vi "errorHandling.vi"() -> ()   [LabVIEW 2014]
uses:
  <vilib>/gmath/statdist.llb/Normal PDF.vi
  <vilib>/gmath/statdist.llb/Poisson Random.vi
  <vilib>/gmath/NI_Gmath.lvlib
panel:
  in  "Normalization 3":dbl
  in  "Normalization 2":dbl
  in  "Normalization 1":dbl
  out "Error State":errorcluster
  out "Waveform Graph":i32[](graph)
  in  "Standard Dev. 3":dbl=5.0 format="%#_13g"
  in  "Mean 3":dbl=25.0 format="%#_13g"
  in  "Standard Dev. 2":dbl=5.0 format="%#_13g"
  in  "Mean 2":dbl=25.0 format="%#_13g"
  in  "Standard Dev. 1":dbl=5.0 format="%#_13g"
  in  "Mean 1":dbl=25.0 format="%#_13g"
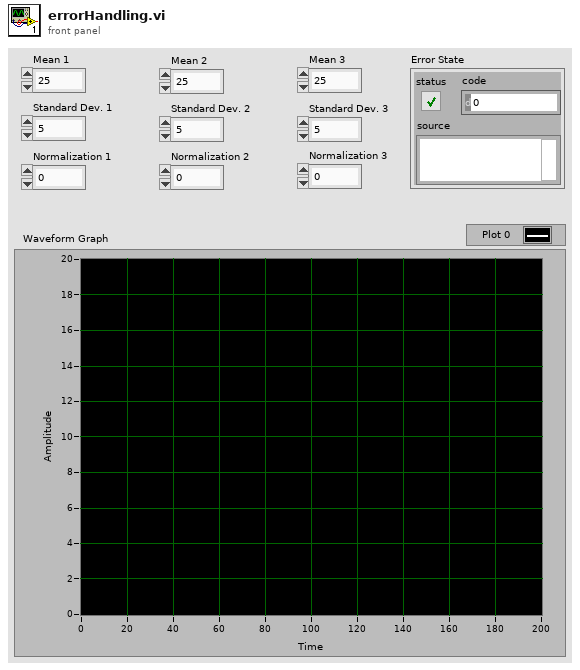
[diagram p1: front panel]
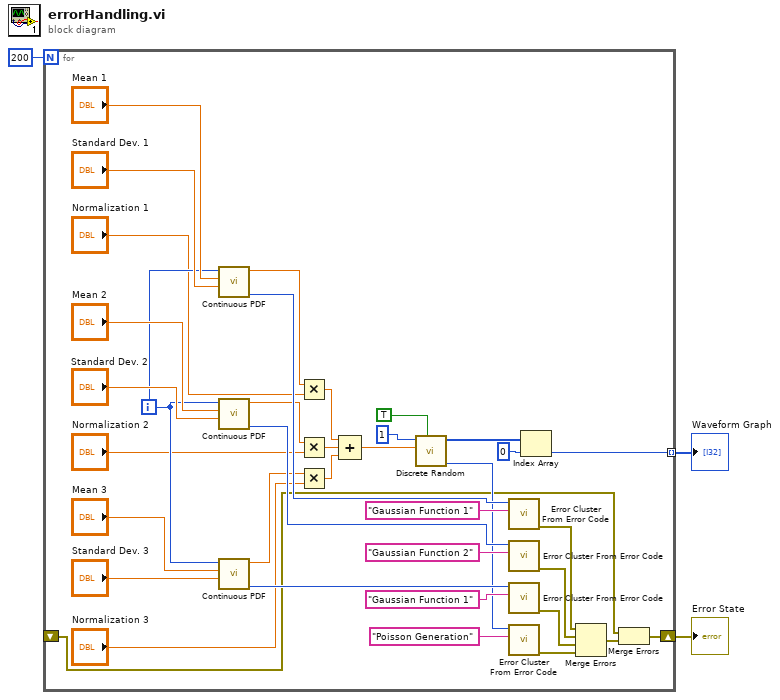
[diagram p0: block diagram]
diagram:
  n1 = for {
    N: 200 -> [_]
    tunnel: [w13] -> w2 mode=indexing
    shift-right: [w17] -> w1
    shift-left: _ -> [w19]
    i -> [w34]
    n2 = call-poly <vilib>:"Continuous PDF.vi"("std"="Standard Dev. 1", "mean"="Mean 1", "x"=w34) -> ("error"=w32:i32, "pdf(x)"=w11:dbl)  [unwired: 7 in]
    n3 = call-poly <vilib>:"Continuous PDF.vi"("std"="Standard Dev. 2", "mean"="Mean 2", "x"=w34) -> ("error"=w30:i32, "pdf(x)"=w8:dbl)  [unwired: 7 in]
    n4 = call-poly <vilib>:"Continuous PDF.vi"("std"="Standard Dev. 3", "mean"="Mean 3", "x"=w34) -> ("error"=w28:i32, "pdf(x)"=w5:dbl)  [unwired: 7 in]
    n5 = Multiply(x=w11, y="Normalization 1") -> (x*y=w10:dbl)
    n6 = Multiply(x=w8, y="Normalization 2") -> (x*y=w7:dbl)
    n7 = Multiply(x=w5, y="Normalization 3") -> (x*y=w4:dbl)
    n8 = Compound Arithmetic op=ADD(w10, w7, w4) -> (w24:dbl)
    n9 = call-poly <vilib>:"Discrete Random.vi"("reset"=TRUE, "lambda"=w24, "samples"=1) -> ("error"=w22:i32, "Poisson random data"=w15:i32[])  [unwired: 7 in]
    n10 = call <vilib>:"Error Cluster From Error Code.vi"("error message (\"\")"="Gaussian Function 1" ("source"), "error code (0)"=w32) -> ("error out"=w27:errorcluster)  [unwired: 7 in]
    n11 = call <vilib>:"Error Cluster From Error Code.vi"("error message (\"\")"="Gaussian Function 2" ("source"), "error code (0)"=w30) -> ("error out"=w26:errorcluster)  [unwired: 7 in]
    n12 = call <vilib>:"Error Cluster From Error Code.vi"("error message (\"\")"="Gaussian Function 1" ("source"), "error code (0)"=w28) -> ("error out"=w25:errorcluster)  [unwired: 7 in]
    n13 = call <vilib>:"Error Cluster From Error Code.vi"("error message (\"\")"="Poisson Generation" ("error message (\"\")"), "error code (0)"=w22) -> ("error out"=w20:errorcluster)  [unwired: 7 in]
    n14 = Index Array(array=w15, index=0) -> (element=w13:i32)
    n15 = Merge Errors(w27, w26, w25, w20) -> (w18:errorcluster)
    n16 = Merge Errors(w19, w18) -> (w17:errorcluster)
  }
  "Waveform Graph" <- w2
  "Error State" <- w1
